vi "RPMToRawUnits.vi"(9 "Gear Ratio":dbl, 10 "RPM":dbl) -> (2 "Raw Units":i32)   [LabVIEW 2019]
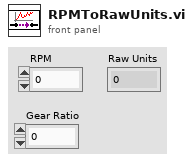
[diagram p1: front panel]
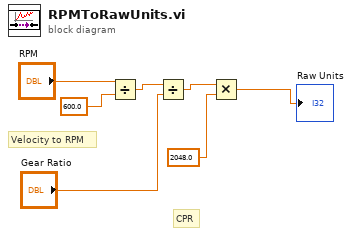
[diagram p0: block diagram]
diagram:
  # "CPR"
  # "Velocity to RPM"
  n1 = Divide(x="RPM", y=600.0) -> (x/y=w5:dbl)
  n2 = Divide(x=w5, y="Gear Ratio") -> (x/y=w3:dbl)
  n3 = Multiply(x=w3, y=2048.0 ("x")) -> (x*y=→"Raw Units":dbl)
